vi "about.vi"   [LabVIEW 2015]
uses:
  ESLSCDLL.dll
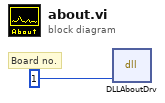
[diagram p0: block diagram]
diagram:
  # "Board no."
  n1 = dll-call lib="C:/Users/Gerhard/Desktop/GS/lv64/1cam/board.vis/ESLSCDLL.dll" fn="DLLAboutDrv"("arg1"=u32 1) -> ()  [unwired: 5 in, 2 out]
